vi "Read DI DAQ Data.vi"(0 "DAQ Node Dict DVR":T1, 1 "DI TaskName":string, 2 "DIStateChangeEv":refnum<user-event>, 5 "DAQ Data Dict DVR":T1, 7 "DI IONames":string[](array[string]), 9 "daqThread DI local Q":refnum<queue>, 11 "error in":errorcluster) -> (4 "DAQ Node Dict DVR out":T1, 6 "DAQ Data Dict DVR out":T1, 15 "error out":errorcluster)   [LabVIEW 2022 SP3, in "DAQ.lvclass"]
doc: "Developed by Kevin Thompson\nkevin@thompsonengineering.net\n\nCopyright 2018-2020\nThompson Engineering, LLC"
uses:
  DAQ.lvclass
  TD local raw DI Data--cluster.ctl
  <vilib>/TELLC/Dynamic CVT API/TD Dynamic CVT DVR--ref.ctl
  DataTypes/TD DAQ DI state change ev.ctl
  DAQ.lvclass/DAQ.ctl
  DataTypes/TD FireDIStateChangeEventTrigger--cluster.ctl
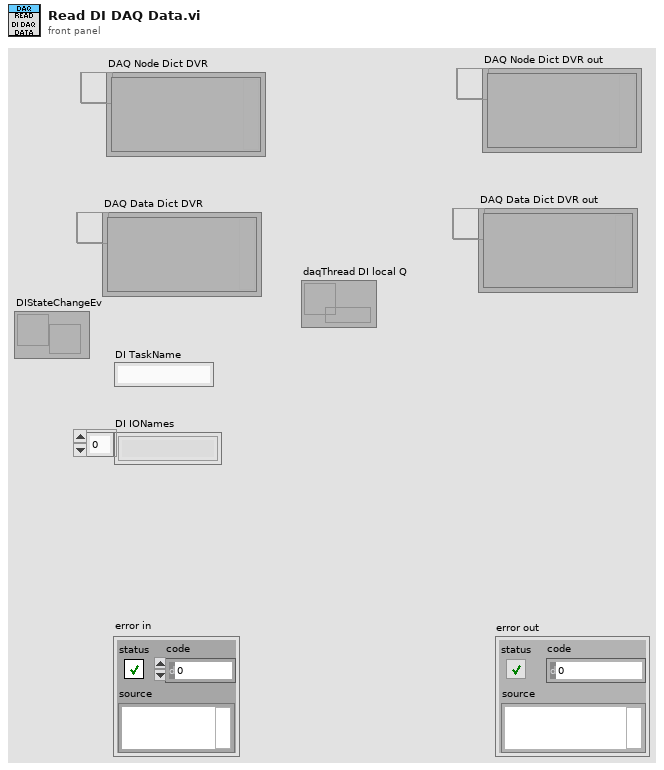
[diagram p1: front panel]
types:
  T1 = typedef "TD Dynamic CVT DVR--ref.ctl" = refnum<data-value>
  T2 = typedef "TD FireDIStateChangeEventTrigger--cluster.ctl" = enum16{"RisingEdge", "FallingEdge", "Both", "Disable"}
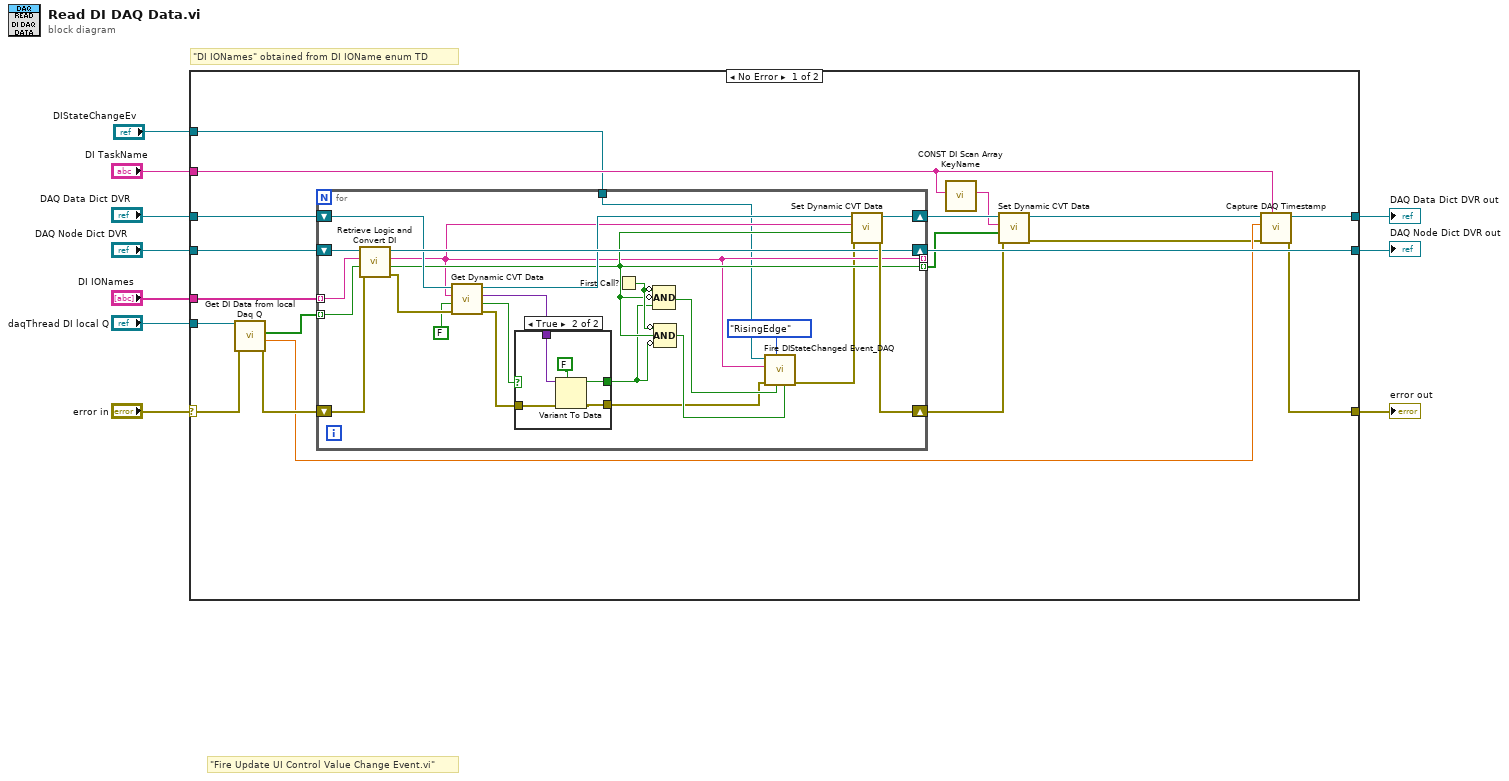
[diagram p0: block diagram]
diagram:
  # "\"Fire Update UI Control Value Change Event.vi\""
  # "\"DI IONames\" obtained from DI IOName enum TD"
  n1 = case shown="No Error" "error in" {
    selector: "error in" -> [w25 w61]
    tunnel: "DI TaskName" -> [w15 _]
    tunnel: "DI IONames" -> [w11 _]
    tunnel: "daqThread DI local Q" -> [w22 _]
    tunnel: "DAQ Data Dict DVR" -> [w29 w62]
    tunnel: [w28 w62] -> w3
    tunnel: [w16 w61] -> w4
    tunnel: "DAQ Node Dict DVR" -> [w27 w60]
    tunnel: [w26 w60] -> w2
    tunnel: "DIStateChangeEv" -> [w13 _]
    frame No Error {
      n2 = call "Get DI Data from local Daq Q.vi"("error in"=w25, "daqThread DI local Q"=w22) -> ("error out"=w23:errorcluster, "timestamp"=w21:dbl, "data"=w24:bool[])  [unwired: 6 in, 1 out]
      n3 = for {
        tunnel: w24 -> [w48] mode=indexing
        tunnel: w11 -> [w47] mode=indexing
        shift-right: [w53] -> w20
        shift-left: w29 -> [w46]
        shift-right: [w52] -> w18
        shift-left: w23 -> [w49]
        shift-right: [w50] -> w26
        shift-left: w27 -> [w51]
        tunnel: [w35] -> _ mode=indexing
        tunnel: [w42] -> w12 mode=indexing
        tunnel: w13 -> [w34]
        n4 = call "Retrieve Logic and Convert DI.vi"("error in (no error)"=w49, "RawValue in"=w48, "IOName"=w47, "DAQ Node Dict DVR"=w51) -> ("error out"=w44:errorcluster, "ConvertedValue Out"=w42:bool, "IOName out"=w35:string, "DAQ Node Dict DVR out"=w50:T1)  [unwired: 4 in]
        n5 = call <vilib>:"Get Dynamic CVT Data.vi"("error in (no error)"=w44, "default value (empty variant)"=FALSE, "DataName"=w35, "dCVT DVR"=w46) -> ("error out"=w38:errorcluster, "found"=w39:bool, "value"=w40:variant, "dCVT DVR out"=w45:T1)  [unwired: 4 in]
        n6 = case shown="True" w39 {
          tunnel: w40 -> [_ w59]
          tunnel: w38 -> [w54 w57]
          tunnel: [w54 w56] -> w31
          tunnel: [_ w55] -> w37
          frame False {
          }
          frame True {
            n7 = Variant To Data(error in=w57, type=FALSE, Variant=w59) -> (data=w55:bool, error out=w56:errorcluster)
          }
        }
        n8 = First Call?() -> (First Call?: T/F=w43:bool)
        n9 = Compound Arithmetic op=AND(invert w43, invert w42, w37) -> (w33:bool)
        n10 = Compound Arithmetic op=AND(invert w43, w42, invert w37) -> (w32:bool)
        n11 = call "Fire DIStateChanged Event_DAQ.vi"("Falling"=w32, "Rising"=w33, "FireEvTrigger"=TD_FireDIStateChangeEventTrigger--cluster."RisingEdge", "error in (no error)"=w31, "Name"=w35, "DIStateChangeEv"=w34) -> ("error out"=w30:errorcluster)  [unwired: 5 in]
        n12 = call <vilib>:"Set Dynamic CVT Data.vi"("error in (no error)"=w30, "value"=w42, "DataName"=w35, "dCVT DVR"=w45) -> ("error out"=w52:errorcluster, "dCVT DVR out"=w53:T1)  [unwired: 5 in, 1 out]
      }
      n13 = call "CONST DI Scan Array KeyName.vi"("DI TaskName"=w15) -> ("DI ScanArray (KeyName)"=w14:string)  [unwired: 10 in]
      n14 = call <vilib>:"Set Dynamic CVT Data.vi"("error in (no error)"=w18, "value"=w12, "DataName"=w14, "dCVT DVR"=w20) -> ("error out"=w17:errorcluster, "dCVT DVR out"=w19:T1)  [unwired: 5 in, 1 out]
      n15 = call "Capture DAQ Timestamp.vi"("DaqData dCVT"=w19, "timestamp in"=w21, "error in (no error)"=w17, "AI TaskName"=w15) -> ("DaqData dCVT out"=w28:T1, "error out"=w16:errorcluster)  [unwired: 4 in, 1 out]
    }
    frame Error {
    }
  }
  "DAQ Data Dict DVR out" <- w3
  "error out" <- w4
  "DAQ Node Dict DVR out" <- w2
